vi "Tester2.vi"() -> ()   [LabVIEW 2015, in "TreeSelectionHierarchal.lvclass"]
doc: "<b> </b> <b> </b>\n©2016 Q Software Innovations, LLC (QSI)\nwritten by Quentin Alldredge\nproduced in LabVIEW 2015\n\nsupport@qsoftwareinnovations.com\nwww.qsoftwareinnovations.com\n\nAll rights reserved.\n\nRedistribution and use in source and binary forms, with or without modification, are permitted provided that the following conditions are met:\n\n * Redistributions of source code must retain the above copyright notice, this list of conditions and the following disclaimer.\n * Redistributions in binary form must reproduce the above copyright notice, this list of conditions and the following disclaimer in the documentation and/or other materials provided with the distribution.\n * Neither the name of Q Software Innovations, LLC. nor the names of its contributors may be used to endorse or promote products derived from this software without specific prior written permission.\n\nTHIS SOFTWARE IS PROVIDED BY THE COPYRIGHT HOLDERS AND CONTRIBUTORS \"AS IS\" AND ANY EXPRESS OR IMPLIED WARRANTIES, INCLUDING, BUT NOT LIMITED TO, THE IMPLIED WARRANTIES OF MERCHANTABILITY AND FITNESS FOR A PARTICULAR PURPOSE ARE DISCLAIMED. IN NO EVENT SHALL THE COPYRIGHT OWNER OR CONTRIBUTORS BE LIABLE FOR ANY DIRECT, INDIRECT, INCIDENTAL, SPECIAL, EXEMPLARY, OR CONSEQUENTIAL DAMAGES (INCLUDING, BUT NOT LIMITED TO, PROCUREMENT OF SUBSTITUTE GOODS OR SERVICES; LOSS OF USE, DATA, OR PROFITS; OR BUSINESS INTERRUPTION) HOWEVER CAUSED AND ON ANY THEORY OF LIABILITY, WHETHER IN CONTRACT, STRICT LIABILITY, OR TORT (INCLUDING NEGLIGENCE OR OTHERWISE) ARISING IN ANY WAY OUT OF THE USE OF THIS SOFTWARE, EVEN IF ADVISED OF THE POSSIBILITY OF SUCH DAMAGE."
uses:
  TreeSelectionHierarchal/TreeSelectionHierarchal.lvclass
panel:
  in  "VI Server Class Heirarchy 2":string(tree)
  in  "VI Server Class Heirarchy":string(tree)
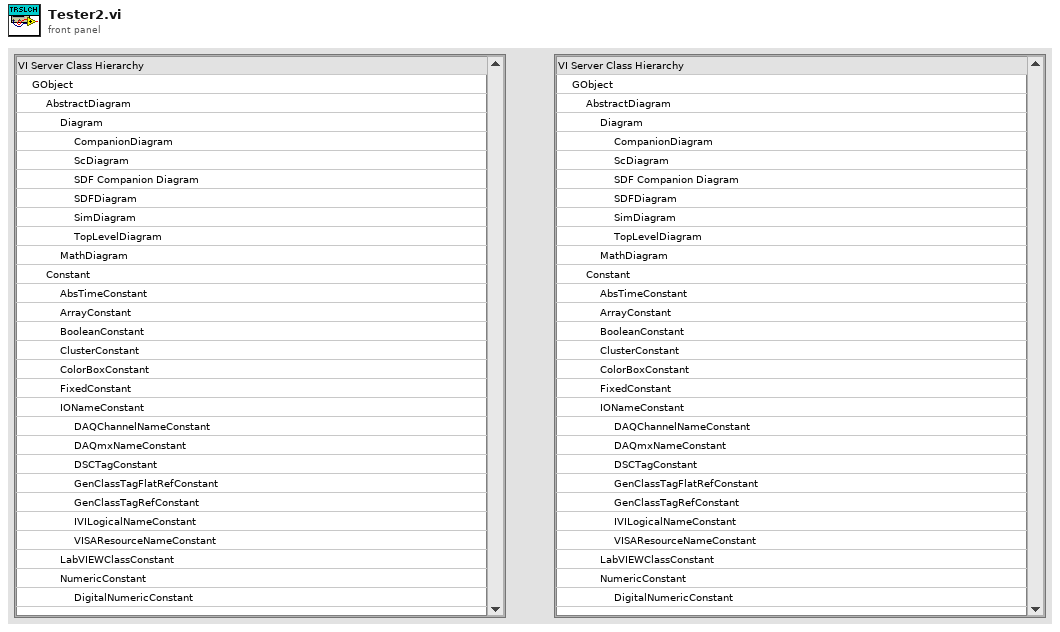
[diagram p1: front panel]
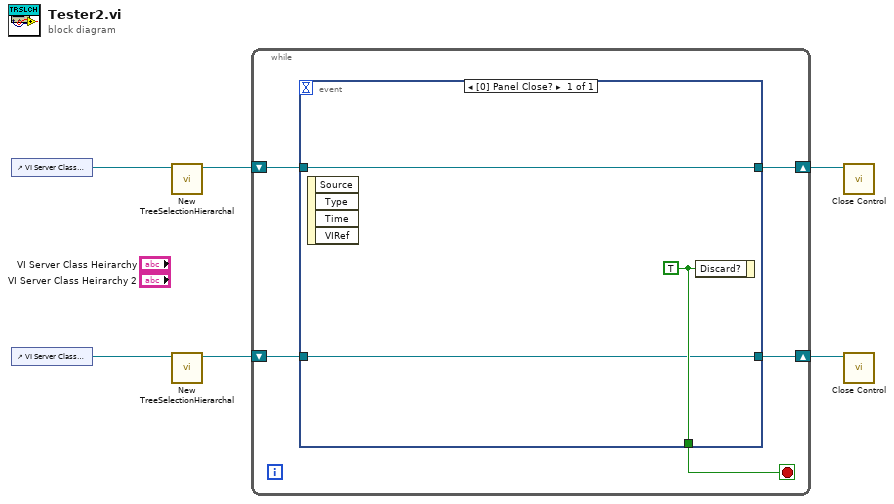
[diagram p0: block diagram]
diagram:
  n1 = control-ref of="VI Server Class Heirarchy"() -> (w5:refnum<vi>)
  n2 = control-ref of="VI Server Class Heirarchy 2"() -> (w2:refnum<vi>)
  n3 = call "New TreeSelectionHierarchal.vi"("Reference"=w5) -> ("TreeSelectionHierarchal out"=w4:refnum<class "TreeSelectionHierarchal.lvclass">)  [unwired: 9 in, 1 out]
  n4 = call "New TreeSelectionHierarchal.vi"("Reference"=w2) -> ("TreeSelectionHierarchal out"=w3:refnum<class "TreeSelectionHierarchal.lvclass">)  [unwired: 9 in, 1 out]
  n5 = while {
    shift-right: [w10] -> w6
    shift-left: w4 -> [w11]
    shift-right: [w8] -> w1
    shift-left: w3 -> [w7]
    stop <- w9 stop-if-true
    n6 = event shown="[0] Panel Close?" {
      selector: _ -> [_]
      dyn-events: _ -> [_]
      timeout: _ -> [_]
      tunnel: w11 -> [w14]
      tunnel: [w14] -> w10
      tunnel: [w13] -> w9
      tunnel: w7 -> [w12]
      tunnel: [w12] -> w8
      event Panel Close? {
        w13 = TRUE ("Discard?")
        n7 = event-data() -> ()  [unwired: 1 in, 4 out]
        n8 = event-data("Discard?"=w13) -> ()  [unwired: 1 in, 1 out]
      }
    }
  }
  n9 = call-dynamic "Close Control.vi"("Control in"=w6) -> ()  [unwired: 9 in, 2 out]
  n10 = call-dynamic "Close Control.vi"("Control in"=w1) -> ()  [unwired: 9 in, 2 out]
